vi "sonar.vi"(8 "error in (no error)":errorcluster, 11 "選擇超音波":enum16{"請選擇超音波", "超音波1", "超音波2", "超音波3", "超音波4"}(ring)) -> (0 "error out":errorcluster, 2 "公分":dbl)   [LabVIEW 2019]
uses:
  <vilib>/Utility/error.llb/Error Cluster From Error Code.vi
  <vilib>/myRIO/Common/Instrument Driver Framework/myRIO v1.0/DIO/vis/myRIO v1.0 Write DIO.vi
  <vilib>/myRIO/Common/Instrument Driver Framework/myRIO v1.0/DIO/vis/myRIO v1.0 Read DIO.vi
  <vilib>/myRIO/Instrument Drivers/Onboard IO/DIO/DIO.lvlib
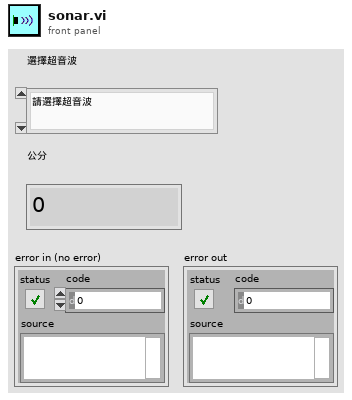
[diagram p1: front panel]
types:
  T1 = typedef "DIO.lvlib/DIO Reference.ctl" = cluster{"myRIO Reference":T2, "DIO Channels List":T6}
  T2 = typedef "myRIO Generic Hardware Reference.ctl" = cluster{"myRIO Model":T3, "myRIO Hardware Reference":T4}
  T3 = typedef "Hardware Version Enum.ctl" = enum16{"Unknown", "myRIO-1900", "myRIO-1950", "roboRIO", "NI ELVIS RIO CM", "ELVIS III"}
  T4 = typedef "myRIO v1.0 Reference.ctl" = cluster{"Generic FPGA Reference":T5, "Allow multiple opens":bool}
  T5 = typedef "Generic FPGA Reference.ctl" = refnum<k20>
  T6 = typedef "DIO Channels List.ctl" = T7[]
  T7 = typedef "DIO Channels Enum.ctl" = enum16{"Not Connected", "C/DIO0", "C/DIO1", "C/DIO2", "C/DIO3", "C/DIO4", "C/DIO5", "C/DIO6", "C/DIO7", "A/DIO0", "A/DIO1", "A/DIO2", "A/DIO3", "A/DIO4", "A/DIO5", "A/DIO6", "A/DIO7", "A/DIO8", "A/DIO9", "A/DIO10", "A/DIO11", "A/DIO12", "A/DIO13", "A/DIO14", "A/DIO15", "A/DIO16", "A/DIO17", "A/DIO18", "A/DIO19", "B/DIO0", "B/DIO1", "B/DIO2", "B/DIO3", "B/DIO4", "B/DIO5", "B/DIO6", "B/DIO7", "B/DIO8", "B/DIO9", "B/DIO10", "B/DIO11", "B/DIO12", "B/DIO13", "B/DIO14", "B/DIO15", "B/DIO16", "B/DIO17", "B/DIO18", "B/DIO19", "LED0", "LED1", "LED2", "LED3", "Button0", "DIO/DIO0", "DIO/DIO1", "DIO/DIO2", "DIO/DIO3", "DIO/DIO4", "DIO/DIO5", "DIO/DIO6", "DIO/DIO7", "DIO/DIO8", "DIO/DIO9", "SPI/CS0", "SPI/CS1", "SPI/CS2", "SPI/CS3", "LED RADIO (Green)", "LED RADIO (Red)", "LED COMM (Green)", "LED COMM (Red)", "LED MODE (Green)", "LED MODE (Red)"}
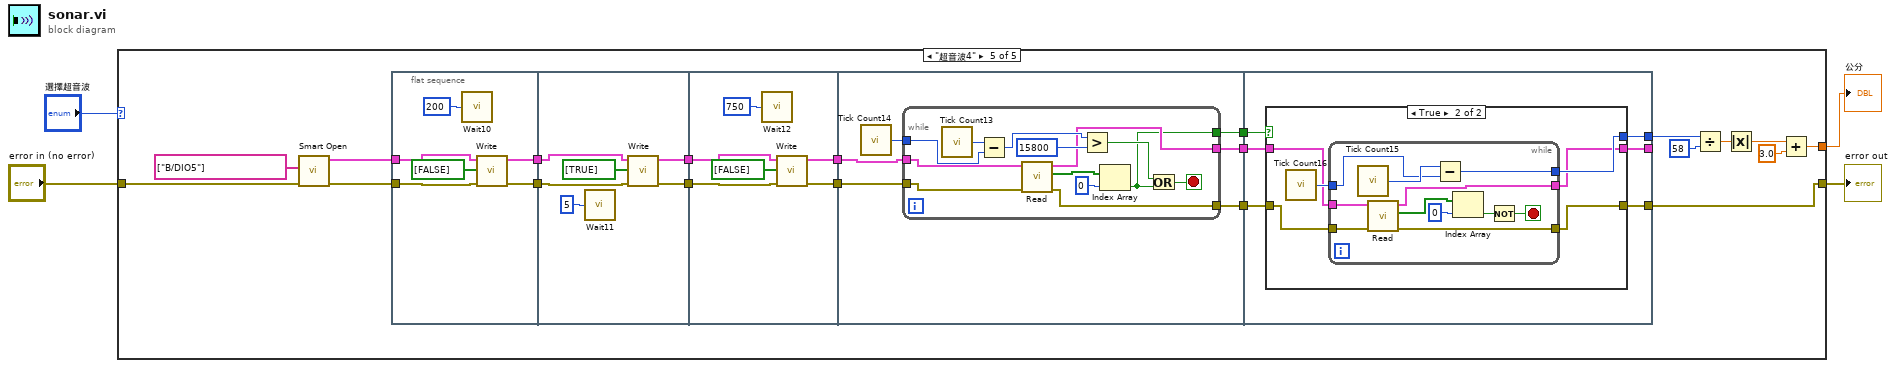
[diagram p0: block diagram]
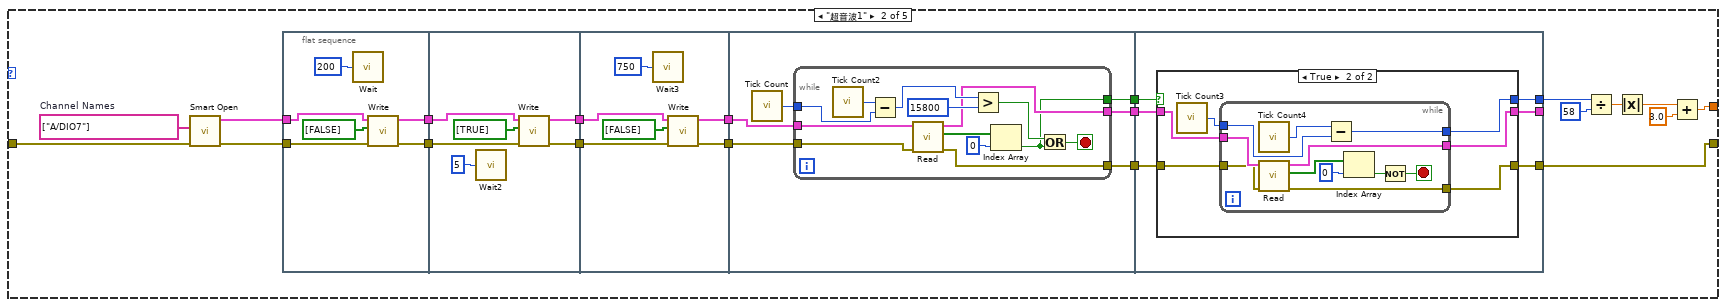
[diagram p3: hidden frame]
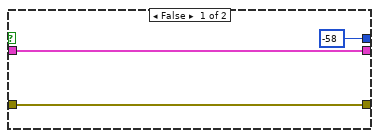
[diagram p4: hidden frame]
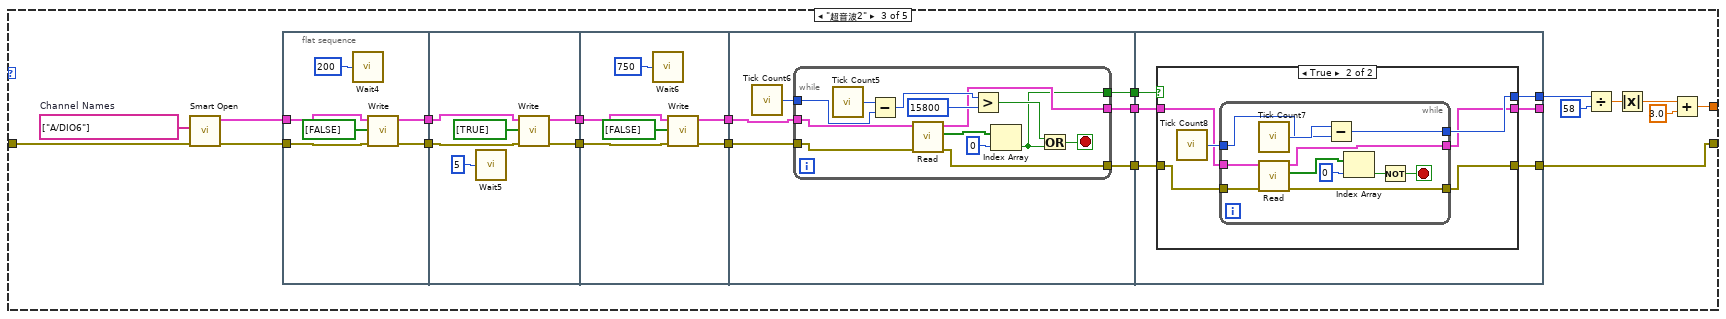
[diagram p5: hidden frame]
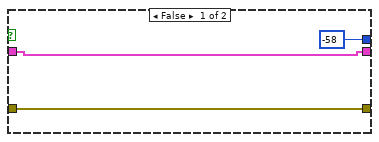
[diagram p6: hidden frame]
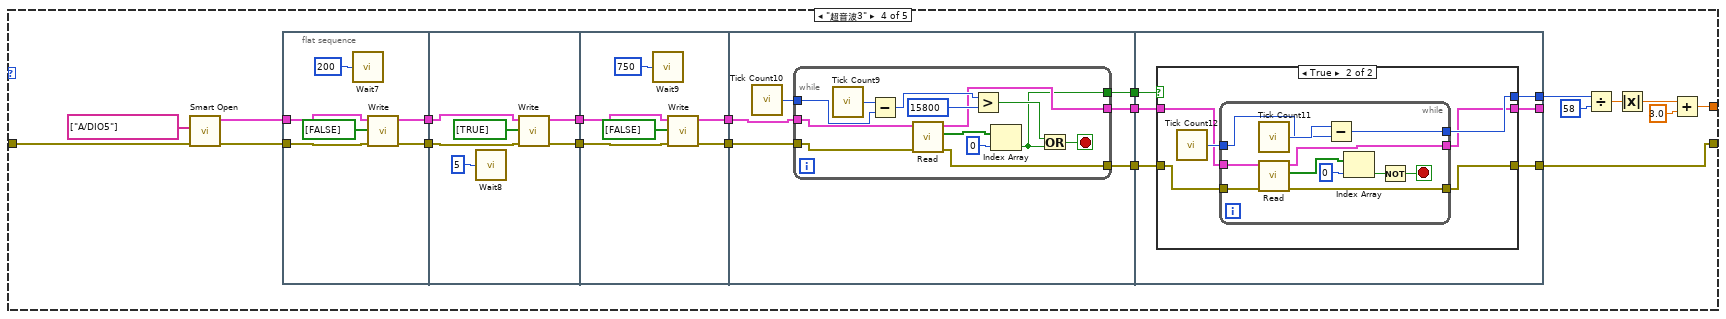
[diagram p7: hidden frame]
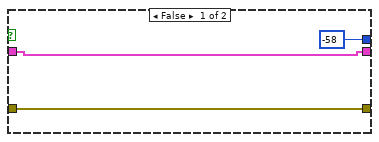
[diagram p8: hidden frame]
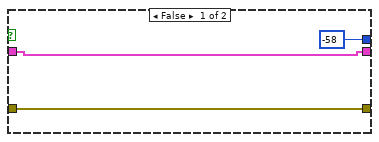
[diagram p9: hidden frame]
diagram:
  n1 = case shown="\"超音波4\"" "選擇超音波" {
    tunnel: "error in (no error)" -> [w5 w16 w94 w177 w260]
    tunnel: [w5 w10 w93 w178 w259] -> w3
    tunnel: [_ w6 w89 w175 w255] -> w1
    frame "請選擇超音波", Default {
    }
    frame "超音波1" {
      w15 = tag[] ["A/DIO7"]  # Channel Names
      n2 = call <vilib>:"Smart Open.vi"("error in (no error)"=w16, "Channel Names"=w15) -> ("error out"=w13:errorcluster, "DIO Ref Out"=w14:T1)  [unwired: 8 in]
      n3 = flat-sequence {
        tunnel: w14 -> [w31]
        tunnel: w13 -> [w30]
        tunnel: [w29] -> w25
        tunnel: [w28] -> w24
        tunnel: w25 -> [w37]
        tunnel: w24 -> [w36]
        tunnel: [w33] -> w23
        tunnel: [w32] -> w22
        tunnel: w23 -> [w42]
        tunnel: w22 -> [w40]
        tunnel: [w39] -> w21
        tunnel: [w38] -> w20
        tunnel: w21 -> [w48]
        tunnel: w20 -> [w47]
        tunnel: [w46] -> w19
        tunnel: [w45] -> w18
        tunnel: [w44] -> w17
        tunnel: w19 -> [w68]
        tunnel: w18 -> [w67]
        tunnel: w17 -> [w66]
        tunnel: [w65] -> _
        tunnel: [w64] -> w10
        tunnel: [w63] -> w12
        frame #0 {
          n4 = call "Wait"("Count(uSec)"=u32 200) -> ()  [unwired: 1 out]
          n5 = call <vilib>:"Write.vi"("error in (no error)"=w30, "Values"=bool[] [FALSE], "DIO Ref In"=w31) -> ("error out"=w28:errorcluster, "DIO Ref Out"=w29:T1)  [unwired: 6 in]
        }
        frame #1 {
          n6 = call "Wait2"("Count(uSec)"=u32 5) -> ()  [unwired: 1 out]
          n7 = call <vilib>:"Write.vi"("error in (no error)"=w36, "Values"=bool[] [TRUE], "DIO Ref In"=w37) -> ("error out"=w32:errorcluster, "DIO Ref Out"=w33:T1)  [unwired: 6 in]
        }
        frame #2 {
          n8 = call "Wait3"("Count(uSec)"=u32 750) -> ()  [unwired: 1 out]
          n9 = call <vilib>:"Write.vi"("error in (no error)"=w40, "Values"=bool[] [FALSE], "DIO Ref In"=w42) -> ("error out"=w38:errorcluster, "DIO Ref Out"=w39:T1)  [unwired: 6 in]
        }
        frame #3 {
          n10 = call "Tick Count"() -> ("Tick Count(uSec)"=w49:u32)
          n11 = while {
            tunnel: w49 -> [w61]
            tunnel: w48 -> [w58]
            tunnel: w47 -> [w57]
            tunnel: [w50] -> w46
            tunnel: [w53] -> w45
            tunnel: [w52] -> w44
            stop <- w54 stop-if-true
            n12 = call "Tick Count2"() -> ("Tick Count(uSec)"=w62:u32)
            n13 = Subtract(x=w62, y=w61) -> (x-y=w60:u32)
            n14 = call <vilib>:"Read.vi"("error in (no error)"=w57, "DIO Ref In"=w58) -> ("error out"=w52:errorcluster, "Values"=w56:bool[], "DIO Ref Out"=w53:T1)  [unwired: 7 in]
            n15 = Greater?(x=w60, y=u32 15800) -> (0:w51:bool)
            n16 = Index Array(array=w56, index=0) -> (element=w50:bool)
            n17 = Or(x=w51, y=w50) -> (x .or. y?=w54:bool)
          }
        }
        frame #4 {
          n18 = case shown="True" w68 {
            tunnel: w67 -> [w71 w76]
            tunnel: w66 -> [w70 w75]
            tunnel: [-58 w74] -> w63
            tunnel: [w71 w73] -> w65
            tunnel: [w70 w72] -> w64
            frame False {
            }
            frame True {
              n19 = call "Tick Count3"() -> ("Tick Count(uSec)"=w77:u32)
              n20 = while {
                tunnel: w77 -> [w87]
                tunnel: w76 -> [w84]
                tunnel: w75 -> [w83]
                tunnel: [w80] -> w74
                tunnel: [w79] -> w73
                tunnel: [w78] -> w72
                stop <- w81 stop-if-true
                n21 = call "Tick Count4"() -> ("Tick Count(uSec)"=w88:u32)
                n22 = call <vilib>:"Read.vi"("error in (no error)"=w83, "DIO Ref In"=w84) -> ("error out"=w78:errorcluster, "Values"=w85:bool[], "DIO Ref Out"=w79:T1)  [unwired: 7 in]
                n23 = Subtract(x=w88, y=w87) -> (x-y=w80:u32)
                n24 = Index Array(array=w85, index=0) -> (element=w82:bool)
                n25 = Not(x=w82) -> (.not. x?=w81:bool)
              }
            }
          }
        }
      }
      n26 = Divide(x=w12, y=u32 58) -> (x/y=w9:dbl)
      n27 = Absolute Value(x=w9) -> (abs(x)=w8:dbl)
      n28 = Add(x=w8, y=3.0) -> (x+y=w6:dbl)
    }
    frame "超音波2" {
      w99 = tag[] ["A/DIO6"]  # Channel Names
      n29 = call <vilib>:"Smart Open.vi"("error in (no error)"=w94, "Channel Names"=w99) -> ("error out"=w97:errorcluster, "DIO Ref Out"=w98:T1)  [unwired: 8 in]
      n30 = flat-sequence {
        tunnel: w98 -> [w114]
        tunnel: w97 -> [w113]
        tunnel: [w112] -> w108
        tunnel: [w111] -> w107
        tunnel: w108 -> [w120]
        tunnel: w107 -> [w119]
        tunnel: [w116] -> w106
        tunnel: [w115] -> w105
        tunnel: w106 -> [w125]
        tunnel: w105 -> [w123]
        tunnel: [w122] -> w104
        tunnel: [w121] -> w103
        tunnel: w104 -> [w131]
        tunnel: w103 -> [w130]
        tunnel: [w129] -> w102
        tunnel: [w128] -> w101
        tunnel: [w127] -> w100
        tunnel: w102 -> [w151]
        tunnel: w101 -> [w150]
        tunnel: w100 -> [w149]
        tunnel: [w148] -> _
        tunnel: [w147] -> w93
        tunnel: [w146] -> w96
        frame #0 {
          n31 = call "Wait4"("Count(uSec)"=u32 200) -> ()  [unwired: 1 out]
          n32 = call <vilib>:"Write.vi"("error in (no error)"=w113, "Values"=bool[] [FALSE], "DIO Ref In"=w114) -> ("error out"=w111:errorcluster, "DIO Ref Out"=w112:T1)  [unwired: 6 in]
        }
        frame #1 {
          n33 = call "Wait5"("Count(uSec)"=u32 5) -> ()  [unwired: 1 out]
          n34 = call <vilib>:"Write.vi"("error in (no error)"=w119, "Values"=bool[] [TRUE], "DIO Ref In"=w120) -> ("error out"=w115:errorcluster, "DIO Ref Out"=w116:T1)  [unwired: 6 in]
        }
        frame #2 {
          n35 = call "Wait6"("Count(uSec)"=u32 750) -> ()  [unwired: 1 out]
          n36 = call <vilib>:"Write.vi"("error in (no error)"=w123, "Values"=bool[] [FALSE], "DIO Ref In"=w125) -> ("error out"=w121:errorcluster, "DIO Ref Out"=w122:T1)  [unwired: 6 in]
        }
        frame #3 {
          n37 = call "Tick Count6"() -> ("Tick Count(uSec)"=w132:u32)
          n38 = while {
            tunnel: w132 -> [w144]
            tunnel: w131 -> [w141]
            tunnel: w130 -> [w140]
            tunnel: [w133] -> w129
            tunnel: [w136] -> w128
            tunnel: [w135] -> w127
            stop <- w137 stop-if-true
            n39 = call "Tick Count5"() -> ("Tick Count(uSec)"=w145:u32)
            n40 = Subtract(x=w145, y=w144) -> (x-y=w143:u32)
            n41 = call <vilib>:"Read.vi"("error in (no error)"=w140, "DIO Ref In"=w141) -> ("error out"=w135:errorcluster, "Values"=w139:bool[], "DIO Ref Out"=w136:T1)  [unwired: 7 in]
            n42 = Greater?(x=w143, y=u32 15800) -> (0:w134:bool)
            n43 = Index Array(array=w139, index=0) -> (element=w133:bool)
            n44 = Or(x=w134, y=w133) -> (x .or. y?=w137:bool)
          }
        }
        frame #4 {
          n45 = case shown="True" w151 {
            tunnel: w150 -> [w154 w159]
            tunnel: w149 -> [w153 w158]
            tunnel: [-58 w157] -> w146
            tunnel: [w154 w156] -> w148
            tunnel: [w153 w155] -> w147
            frame False {
            }
            frame True {
              n46 = call "Tick Count8"() -> ("Tick Count(uSec)"=w160:u32)
              n47 = while {
                tunnel: w160 -> [w170]
                tunnel: w159 -> [w167]
                tunnel: w158 -> [w166]
                tunnel: [w163] -> w157
                tunnel: [w162] -> w156
                tunnel: [w161] -> w155
                stop <- w164 stop-if-true
                n48 = call "Tick Count7"() -> ("Tick Count(uSec)"=w171:u32)
                n49 = call <vilib>:"Read.vi"("error in (no error)"=w166, "DIO Ref In"=w167) -> ("error out"=w161:errorcluster, "Values"=w168:bool[], "DIO Ref Out"=w162:T1)  [unwired: 7 in]
                n50 = Subtract(x=w171, y=w170) -> (x-y=w163:u32)
                n51 = Index Array(array=w168, index=0) -> (element=w165:bool)
                n52 = Not(x=w165) -> (.not. x?=w164:bool)
              }
            }
          }
        }
      }
      n53 = Divide(x=w96, y=u32 58) -> (x/y=w92:dbl)
      n54 = Absolute Value(x=w92) -> (abs(x)=w91:dbl)
      n55 = Add(x=w91, y=3.0) -> (x+y=w89:dbl)
    }
    frame "超音波3" {
      n56 = call <vilib>:"Smart Open.vi"("error in (no error)"=w177, "Channel Names"=tag[] ["A/DIO5"]) -> ("error out"=w181:errorcluster, "DIO Ref Out"=w182:T1)  [unwired: 8 in]
      n57 = flat-sequence {
        tunnel: w182 -> [w197]
        tunnel: w181 -> [w196]
        tunnel: [w195] -> w191
        tunnel: [w194] -> w190
        tunnel: w191 -> [w203]
        tunnel: w190 -> [w202]
        tunnel: [w199] -> w189
        tunnel: [w198] -> w188
        tunnel: w189 -> [w208]
        tunnel: w188 -> [w206]
        tunnel: [w205] -> w187
        tunnel: [w204] -> w186
        tunnel: w187 -> [w214]
        tunnel: w186 -> [w213]
        tunnel: [w212] -> w185
        tunnel: [w211] -> w184
        tunnel: [w210] -> w183
        tunnel: w185 -> [w234]
        tunnel: w184 -> [w233]
        tunnel: w183 -> [w232]
        tunnel: [w231] -> _
        tunnel: [w230] -> w178
        tunnel: [w229] -> w180
        frame #0 {
          n58 = call "Wait7"("Count(uSec)"=u32 200) -> ()  [unwired: 1 out]
          n59 = call <vilib>:"Write.vi"("error in (no error)"=w196, "Values"=bool[] [FALSE], "DIO Ref In"=w197) -> ("error out"=w194:errorcluster, "DIO Ref Out"=w195:T1)  [unwired: 6 in]
        }
        frame #1 {
          n60 = call "Wait8"("Count(uSec)"=u32 5) -> ()  [unwired: 1 out]
          n61 = call <vilib>:"Write.vi"("error in (no error)"=w202, "Values"=bool[] [TRUE], "DIO Ref In"=w203) -> ("error out"=w198:errorcluster, "DIO Ref Out"=w199:T1)  [unwired: 6 in]
        }
        frame #2 {
          n62 = call "Wait9"("Count(uSec)"=u32 750) -> ()  [unwired: 1 out]
          n63 = call <vilib>:"Write.vi"("error in (no error)"=w206, "Values"=bool[] [FALSE], "DIO Ref In"=w208) -> ("error out"=w204:errorcluster, "DIO Ref Out"=w205:T1)  [unwired: 6 in]
        }
        frame #3 {
          n64 = call "Tick Count10"() -> ("Tick Count(uSec)"=w215:u32)
          n65 = while {
            tunnel: w215 -> [w227]
            tunnel: w214 -> [w224]
            tunnel: w213 -> [w223]
            tunnel: [w216] -> w212
            tunnel: [w219] -> w211
            tunnel: [w218] -> w210
            stop <- w220 stop-if-true
            n66 = call "Tick Count9"() -> ("Tick Count(uSec)"=w228:u32)
            n67 = Subtract(x=w228, y=w227) -> (x-y=w226:u32)
            n68 = call <vilib>:"Read.vi"("error in (no error)"=w223, "DIO Ref In"=w224) -> ("error out"=w218:errorcluster, "Values"=w222:bool[], "DIO Ref Out"=w219:T1)  [unwired: 7 in]
            n69 = Greater?(x=w226, y=u32 15800) -> (0:w217:bool)
            n70 = Index Array(array=w222, index=0) -> (element=w216:bool)
            n71 = Or(x=w217, y=w216) -> (x .or. y?=w220:bool)
          }
        }
        frame #4 {
          n72 = case shown="True" w234 {
            tunnel: w233 -> [w237 w242]
            tunnel: w232 -> [w236 w241]
            tunnel: [-58 w240] -> w229
            tunnel: [w237 w239] -> w231
            tunnel: [w236 w238] -> w230
            frame False {
            }
            frame True {
              n73 = call "Tick Count12"() -> ("Tick Count(uSec)"=w243:u32)
              n74 = while {
                tunnel: w243 -> [w253]
                tunnel: w242 -> [w250]
                tunnel: w241 -> [w249]
                tunnel: [w246] -> w240
                tunnel: [w245] -> w239
                tunnel: [w244] -> w238
                stop <- w247 stop-if-true
                n75 = call "Tick Count11"() -> ("Tick Count(uSec)"=w254:u32)
                n76 = call <vilib>:"Read.vi"("error in (no error)"=w249, "DIO Ref In"=w250) -> ("error out"=w244:errorcluster, "Values"=w251:bool[], "DIO Ref Out"=w245:T1)  [unwired: 7 in]
                n77 = Subtract(x=w254, y=w253) -> (x-y=w246:u32)
                n78 = Index Array(array=w251, index=0) -> (element=w248:bool)
                n79 = Not(x=w248) -> (.not. x?=w247:bool)
              }
            }
          }
        }
      }
      n80 = Divide(x=w180, y=u32 58) -> (x/y=w173:dbl)
      n81 = Absolute Value(x=w173) -> (abs(x)=w172:dbl)
      n82 = Add(x=w172, y=3.0) -> (x+y=w175:dbl)
    }
    frame "超音波4" {
      n83 = call <vilib>:"Smart Open.vi"("error in (no error)"=w260, "Channel Names"=tag[] ["B/DIO5"]) -> ("error out"=w264:errorcluster, "DIO Ref Out"=w265:T1)  [unwired: 8 in]
      n84 = flat-sequence {
        tunnel: w265 -> [w280]
        tunnel: w264 -> [w279]
        tunnel: [w278] -> w274
        tunnel: [w277] -> w273
        tunnel: w274 -> [w286]
        tunnel: w273 -> [w285]
        tunnel: [w282] -> w272
        tunnel: [w281] -> w271
        tunnel: w272 -> [w291]
        tunnel: w271 -> [w289]
        tunnel: [w288] -> w270
        tunnel: [w287] -> w269
        tunnel: w270 -> [w297]
        tunnel: w269 -> [w296]
        tunnel: [w295] -> w268
        tunnel: [w294] -> w267
        tunnel: [w293] -> w266
        tunnel: w268 -> [w317]
        tunnel: w267 -> [w316]
        tunnel: w266 -> [w315]
        tunnel: [w314] -> _
        tunnel: [w313] -> w259
        tunnel: [w312] -> w263
        frame #0 {
          n85 = call "Wait10"("Count(uSec)"=u32 200) -> ()  [unwired: 1 out]
          n86 = call <vilib>:"Write.vi"("error in (no error)"=w279, "Values"=bool[] [FALSE], "DIO Ref In"=w280) -> ("error out"=w277:errorcluster, "DIO Ref Out"=w278:T1)  [unwired: 6 in]
        }
        frame #1 {
          n87 = call "Wait11"("Count(uSec)"=u32 5) -> ()  [unwired: 1 out]
          n88 = call <vilib>:"Write.vi"("error in (no error)"=w285, "Values"=bool[] [TRUE], "DIO Ref In"=w286) -> ("error out"=w281:errorcluster, "DIO Ref Out"=w282:T1)  [unwired: 6 in]
        }
        frame #2 {
          n89 = call "Wait12"("Count(uSec)"=u32 750) -> ()  [unwired: 1 out]
          n90 = call <vilib>:"Write.vi"("error in (no error)"=w289, "Values"=bool[] [FALSE], "DIO Ref In"=w291) -> ("error out"=w287:errorcluster, "DIO Ref Out"=w288:T1)  [unwired: 6 in]
        }
        frame #3 {
          n91 = call "Tick Count14"() -> ("Tick Count(uSec)"=w298:u32)
          n92 = while {
            tunnel: w298 -> [w310]
            tunnel: w297 -> [w307]
            tunnel: w296 -> [w306]
            tunnel: [w299] -> w295
            tunnel: [w302] -> w294
            tunnel: [w301] -> w293
            stop <- w303 stop-if-true
            n93 = call "Tick Count13"() -> ("Tick Count(uSec)"=w311:u32)
            n94 = Subtract(x=w311, y=w310) -> (x-y=w309:u32)
            n95 = call <vilib>:"Read.vi"("error in (no error)"=w306, "DIO Ref In"=w307) -> ("error out"=w301:errorcluster, "Values"=w305:bool[], "DIO Ref Out"=w302:T1)  [unwired: 7 in]
            n96 = Greater?(x=w309, y=u32 15800) -> (0:w300:bool)
            n97 = Index Array(array=w305, index=0) -> (element=w299:bool)
            n98 = Or(x=w300, y=w299) -> (x .or. y?=w303:bool)
          }
        }
        frame #4 {
          n99 = case shown="True" w317 {
            tunnel: w316 -> [w320 w325]
            tunnel: w315 -> [w319 w324]
            tunnel: [-58 w323] -> w312
            tunnel: [w320 w322] -> w314
            tunnel: [w319 w321] -> w313
            frame False {
            }
            frame True {
              n100 = call "Tick Count16"() -> ("Tick Count(uSec)"=w326:u32)
              n101 = while {
                tunnel: w326 -> [w336]
                tunnel: w325 -> [w333]
                tunnel: w324 -> [w332]
                tunnel: [w329] -> w323
                tunnel: [w328] -> w322
                tunnel: [w327] -> w321
                stop <- w330 stop-if-true
                n102 = call "Tick Count15"() -> ("Tick Count(uSec)"=w337:u32)
                n103 = call <vilib>:"Read.vi"("error in (no error)"=w332, "DIO Ref In"=w333) -> ("error out"=w327:errorcluster, "Values"=w334:bool[], "DIO Ref Out"=w328:T1)  [unwired: 7 in]
                n104 = Subtract(x=w337, y=w336) -> (x-y=w329:u32)
                n105 = Index Array(array=w334, index=0) -> (element=w331:bool)
                n106 = Not(x=w331) -> (.not. x?=w330:bool)
              }
            }
          }
        }
      }
      n107 = Divide(x=w263, y=u32 58) -> (x/y=w258:dbl)
      n108 = Absolute Value(x=w258) -> (abs(x)=w256:dbl)
      n109 = Add(x=w256, y=3.0) -> (x+y=w255:dbl)
    }
  }
  "error out" <- w3
  "公分" <- w1
